vi "仪器参数设置.vi"(11 "仪器参数设置":T2 {"单位" items=["ug/L", "mg/L"]}) -> (3 "仪器参数设置输出":T1 {"单位" items=["ug/L", "mg/L"]})   [LabVIEW 2016]
uses:
  <vilib>/Utility/miscctls.llb/LVPointTypeDef.ctl
panel:
  in  "水样检出限":cluster{"检出限":dbl, "随机值下限":dbl, "随机值上限":dbl}={"检出限"=0.5, "随机值下限"=0.5, "随机值上限"=1.0}
  in  "锁定按钮":bool
  in  "单位":enum16{"ug/L", "mg/L"}(ring)
  in  "标样校准时间":timestamp
  in  "二次多项式系数":dbl
  in  "线性相关系数":dbl
  in  "测量信号值":dbl
  in  "测量检出限":dbl
  in  "曲线斜率":dbl
  in  "曲线截距":dbl
  in  "空白校准时间":timestamp
  in  "消解时长":dbl
  in  "消解温度":dbl
  in  "测量间隔":dbl
  in  "测量精度":dbl
  in  "测量量程":dbl
  in  "取消":bool
  in  "确定":bool
  # "仪器参数设置"
  # "CODMn"
  # "监测参数"
  # "黑色框参数需要手动输入\n灰色框参数自动读取不需要手动输入"
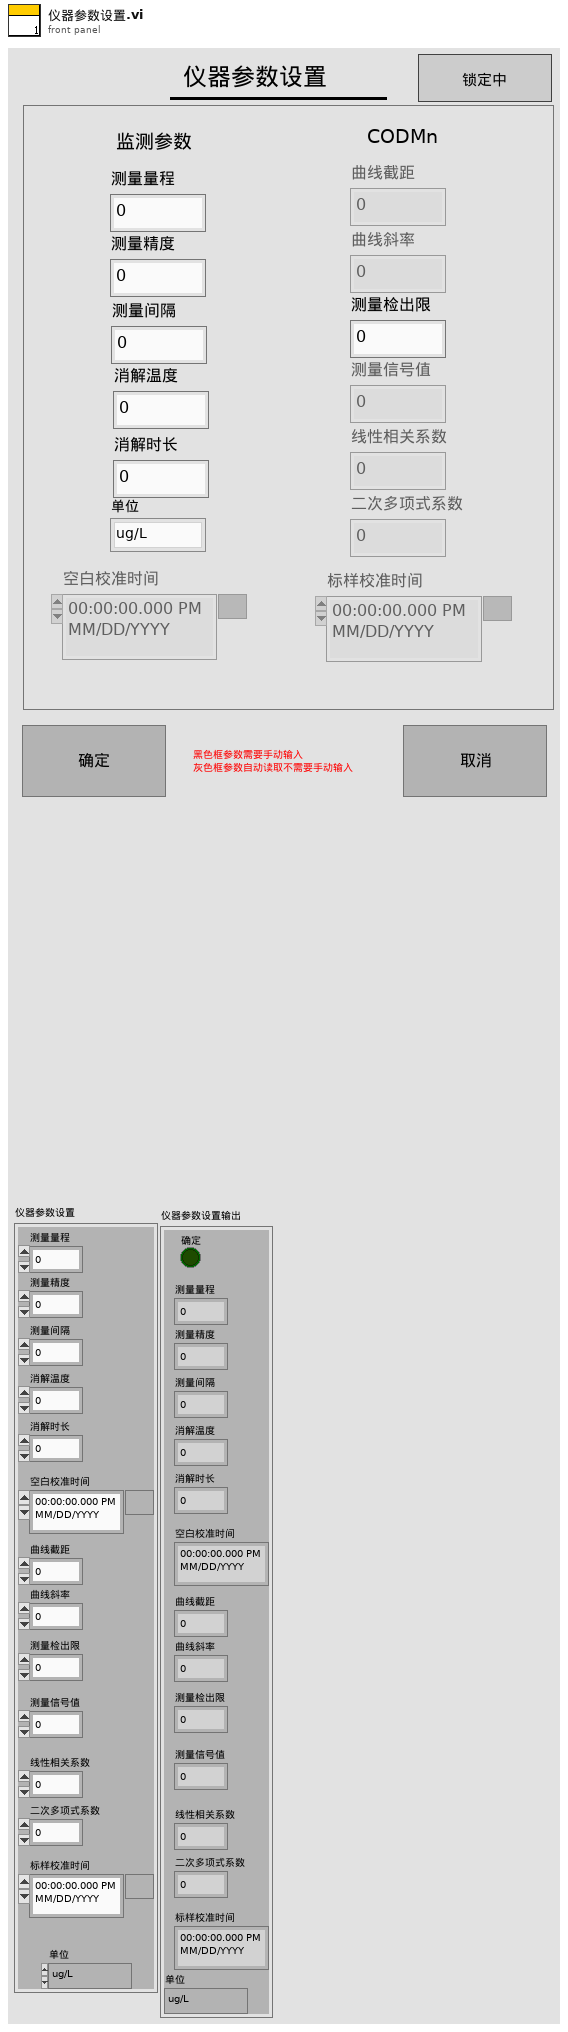
[diagram p1: front panel]
types:
  T1 = cluster{"确定":bool, "测量量程":dbl, "测量精度":dbl, "测量间隔":dbl, "消解温度":dbl, "消解时长":dbl, "空白校准时间":timestamp, "曲线截距":dbl, "曲线斜率":dbl, "测量检出限":dbl, "测量信号值":dbl, "线性相关系数":dbl, "二次多项式系数":dbl, "标样校准时间":timestamp, "单位":u16}
  T2 = cluster{"测量量程":dbl, "测量精度":dbl, "测量间隔":dbl, "消解温度":dbl, "消解时长":dbl, "空白校准时间":timestamp, "曲线截距":dbl, "曲线斜率":dbl, "测量检出限":dbl, "测量信号值":dbl, "线性相关系数":dbl, "二次多项式系数":dbl, "标样校准时间":timestamp, "单位":u16}
  T3 = typedef "LVPointTypeDef.ctl" = cluster{"Horizontal":i16, "Vertical":i16}
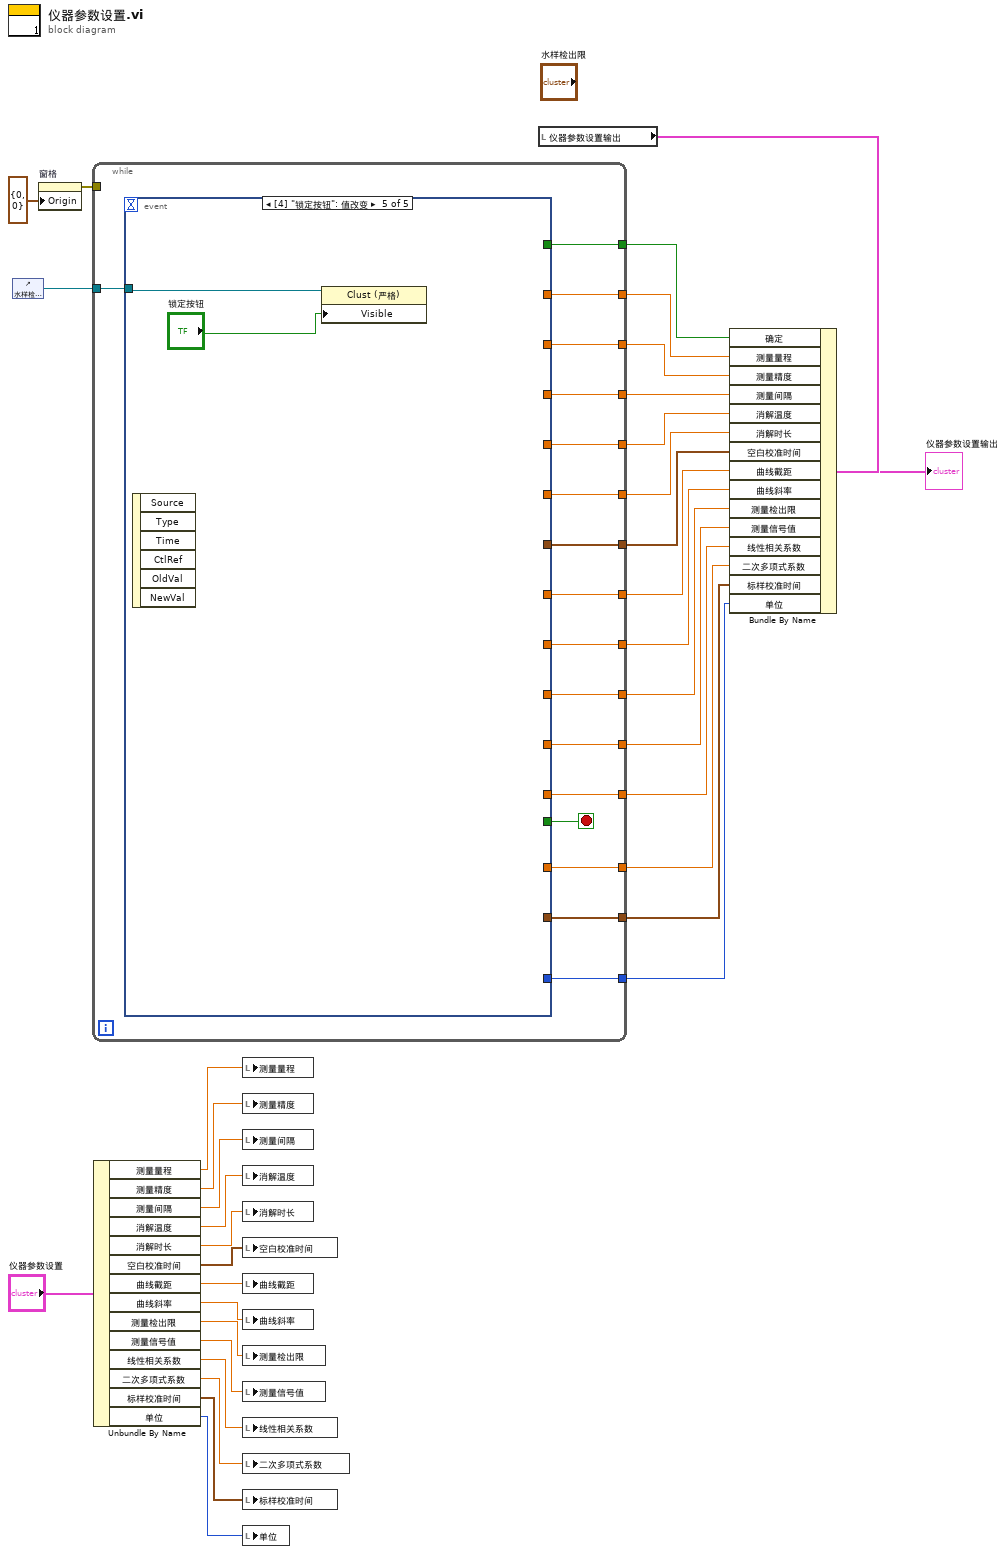
[diagram p0: block diagram]
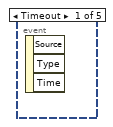
[diagram p2: hidden frame]
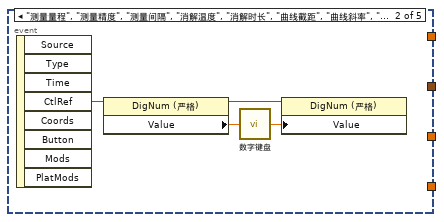
[diagram p3: hidden frame]
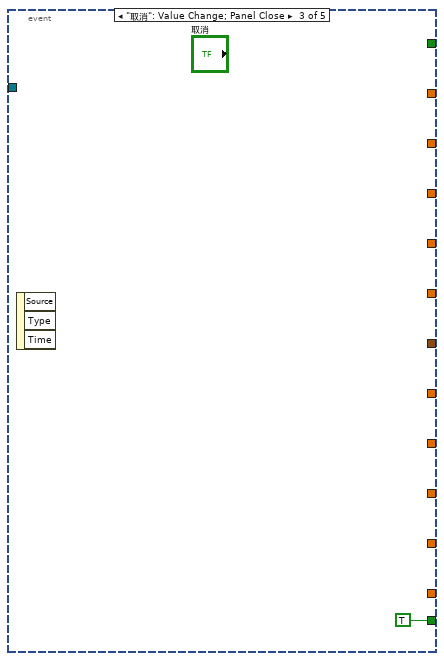
[diagram p4: hidden frame]
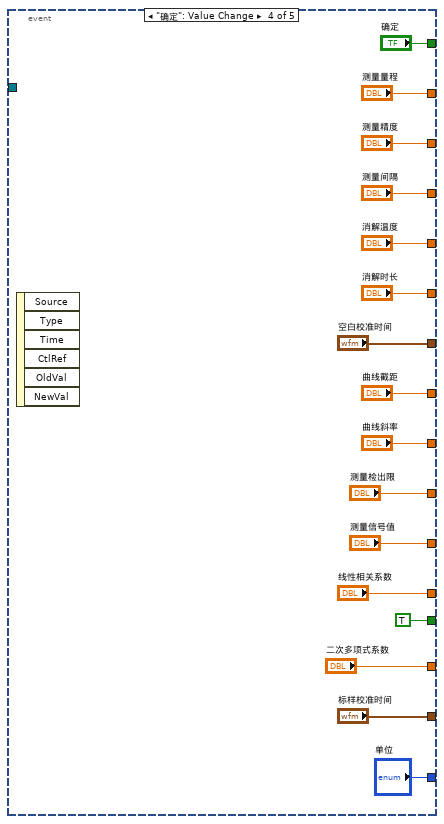
[diagram p5: hidden frame]
diagram:
  n1 = control-ref of="水样检出限"() -> (w1:refnum<vi>)
  n2 = property on="窗格" class="Pane"("Origin"=T3 {"Horizontal"=0, "Vertical"=0} ("原点")) -> (error out=w34:errorcluster)  [unwired: 2 in, 1 out]
  n3 = while {
    tunnel: w34 -> [_]
    tunnel: [w51] -> w33
    tunnel: [w50] -> w29
    tunnel: [w49] -> w28
    tunnel: [w48] -> w27
    tunnel: [w47] -> w26
    tunnel: [w46] -> w25
    tunnel: [w45] -> w24
    tunnel: [w44] -> w23
    tunnel: [w43] -> w22
    tunnel: [w42] -> w21
    tunnel: [w41] -> w20
    tunnel: [w40] -> w19
    tunnel: [w39] -> w18
    tunnel: [w38] -> w17
    tunnel: [w37] -> w2
    tunnel: w1 -> [w36]
    stop <- w52 stop-if-true
    n4 = event shown="[4] \"锁定按钮\": 值改变" {
      selector: _ -> [_ _ _ _ _]
      dyn-events: _ -> [_ _ _ _ _]
      timeout: _ -> [_ _ _ _ _]
      tunnel: [_ _ TRUE TRUE _] -> w52
      tunnel: [_ _ _ "确定" _] -> w51
      tunnel: [_ _ _ "标样校准时间" _] -> w50
      tunnel: [_ _ _ "二次多项式系数" _] -> w49
      tunnel: [_ _ _ "线性相关系数" _] -> w48
      tunnel: [_ _ _ "测量信号值" _] -> w47
      tunnel: [_ _ _ "测量检出限" _] -> w46
      tunnel: [_ _ _ "曲线斜率" _] -> w45
      tunnel: [_ _ _ "曲线截距" _] -> w44
      tunnel: [_ _ _ "空白校准时间" _] -> w43
      tunnel: [_ _ _ "消解时长" _] -> w42
      tunnel: [_ _ _ "消解温度" _] -> w41
      tunnel: [_ _ _ "测量间隔" _] -> w40
      tunnel: [_ _ _ "测量精度" _] -> w39
      tunnel: [_ _ _ "测量量程" _] -> w38
      tunnel: [_ _ _ "单位" _] -> w37
      tunnel: w36 -> [_ _ _ _ w75]
      event Timeout {
        n5 = event-data() -> ()  [unwired: 1 in, 3 out]
      }
      event "测量量程", "测量精度", "测量间隔", "消解温度", "消解时长", "曲线截距", "曲线斜率", "测量检出限", "测量信号值", "线性相关系数", "二次多项式系数": Mouse Down {
        n6 = event-data() -> ("CtlRef"=w53:refnum<vi>)  [unwired: 1 in, 7 out]
        n7 = property class="DigNum (严格)"(reference=w53) -> (reference out=w55:refnum<vi>, "Value"=w56:dbl)  [unwired: 1 in, 1 out]
        n8 = call "数字键盘.vi"("OldNumber"=w56) -> ("NewNumber"=w54:sgl)
        n9 = property class="DigNum (严格)"(reference=w55, "Value"=w54) -> ()  [unwired: 1 in, 2 out]
      }
      event "取消": Value Change; Panel Close {
        n10 = event-data() -> ()  [unwired: 1 in, 3 out]
      }
      event "确定": Value Change {
        n11 = event-data() -> ()  [unwired: 1 in, 6 out]
      }
      event "锁定按钮": Value Change {
        n12 = event-data() -> ()  [unwired: 1 in, 6 out]
        n13 = property class="Clust (严格)"(reference=w75, "Visible"="锁定按钮") -> ()  [unwired: 1 in, 2 out]
      }
    }
  }
  n14 = Unbundle By Name("仪器参数设置") -> ("测量量程"=w16:dbl, "测量精度"=w15:dbl, "测量间隔"=w14:dbl, "消解温度"=w13:dbl, "消解时长"=w12:dbl, "空白校准时间"=w11:timestamp, "曲线截距"=w10:dbl, "曲线斜率"=w9:dbl, "测量检出限"=w8:dbl, "测量信号值"=w7:dbl, "线性相关系数"=w6:dbl, "二次多项式系数"=w5:dbl, "标样校准时间"=w4:timestamp, "单位"=w3:u16)
  n15 = local write "测量量程"(w16) -> ()
  n16 = local write "测量精度"(w15) -> ()
  n17 = local write "测量间隔"(w14) -> ()
  n18 = local write "消解温度"(w13) -> ()
  n19 = local write "消解时长"(w12) -> ()
  n20 = local write "空白校准时间"(w11) -> ()
  n21 = local write "曲线截距"(w10) -> ()
  n22 = local write "曲线斜率"(w9) -> ()
  n23 = local write "测量检出限"(w8) -> ()
  n24 = local write "测量信号值"(w7) -> ()
  n25 = local write "线性相关系数"(w6) -> ()
  n26 = local write "二次多项式系数"(w5) -> ()
  n27 = local write "标样校准时间"(w4) -> ()
  n28 = local write "单位"(w3) -> ()
  n29 = local read "仪器参数设置输出"() -> (w31:T1)
  n30 = Bundle By Name(cluster=w31, "确定"=w33, "测量量程"=w17, "测量精度"=w18, "测量间隔"=w19, "消解温度"=w20, "消解时长"=w21, "空白校准时间"=w22, "曲线截距"=w23, "曲线斜率"=w24, "测量检出限"=w25, "测量信号值"=w26, "线性相关系数"=w27, "二次多项式系数"=w28, "标样校准时间"=w29, "单位"=w2) -> (→"仪器参数设置输出":T1)
